vi "App3_measure_voltage_battery.vi"() -> ()   [LabVIEW 2015]
uses:
  <vilib>/DAQmx/read.llb/DAQmx Read (Analog DBL 1Chan 1Samp).vi
  <vilib>/DAQmx/read.llb/DAQmx Read (Analog Wfm 1Chan NSamp).vi
  <vilib>/DAQmx/miscellaneous.llb/DAQmx Fill In Error Info.vi
panel:
  out "error out":errorcluster
  in  "task out":refnum<k21>
  out "Button 2":u16
  out "Waveform Chart 2":waveform(dbl)
  out "Button":u16
  in  "Tab Control":T1(tab)
  out "min value":dbl
  out "max value":dbl
  out "Delta(s)":dbl
  in  "Zero":bool
  out "Average":dbl
  in  "mA/uA":bool
  out "Waveform Graph":waveform(dbl)(graph)
  in  "uA/mA":bool=TRUE
  out "Waveform Graph 2":waveform(dbl)(graph)
  out "Average (uA)":dbl caption="Average (mV)"
  in  "PAUSE":bool
  out "Vbat":dbl
  out "Waveform Chart":dbl(graph)
  in  "Number of samples uC Board":i32=10000
  in  "USB DAQ":tag="Dev1"
  out "Waveform Chart 3":dbl(graph)
  in  "file List":i32(listbox)
  out "2D Picture":picture
  # "FW Validation - Current Tracking V1.0"
  # "For uC Board: 20kS/s"
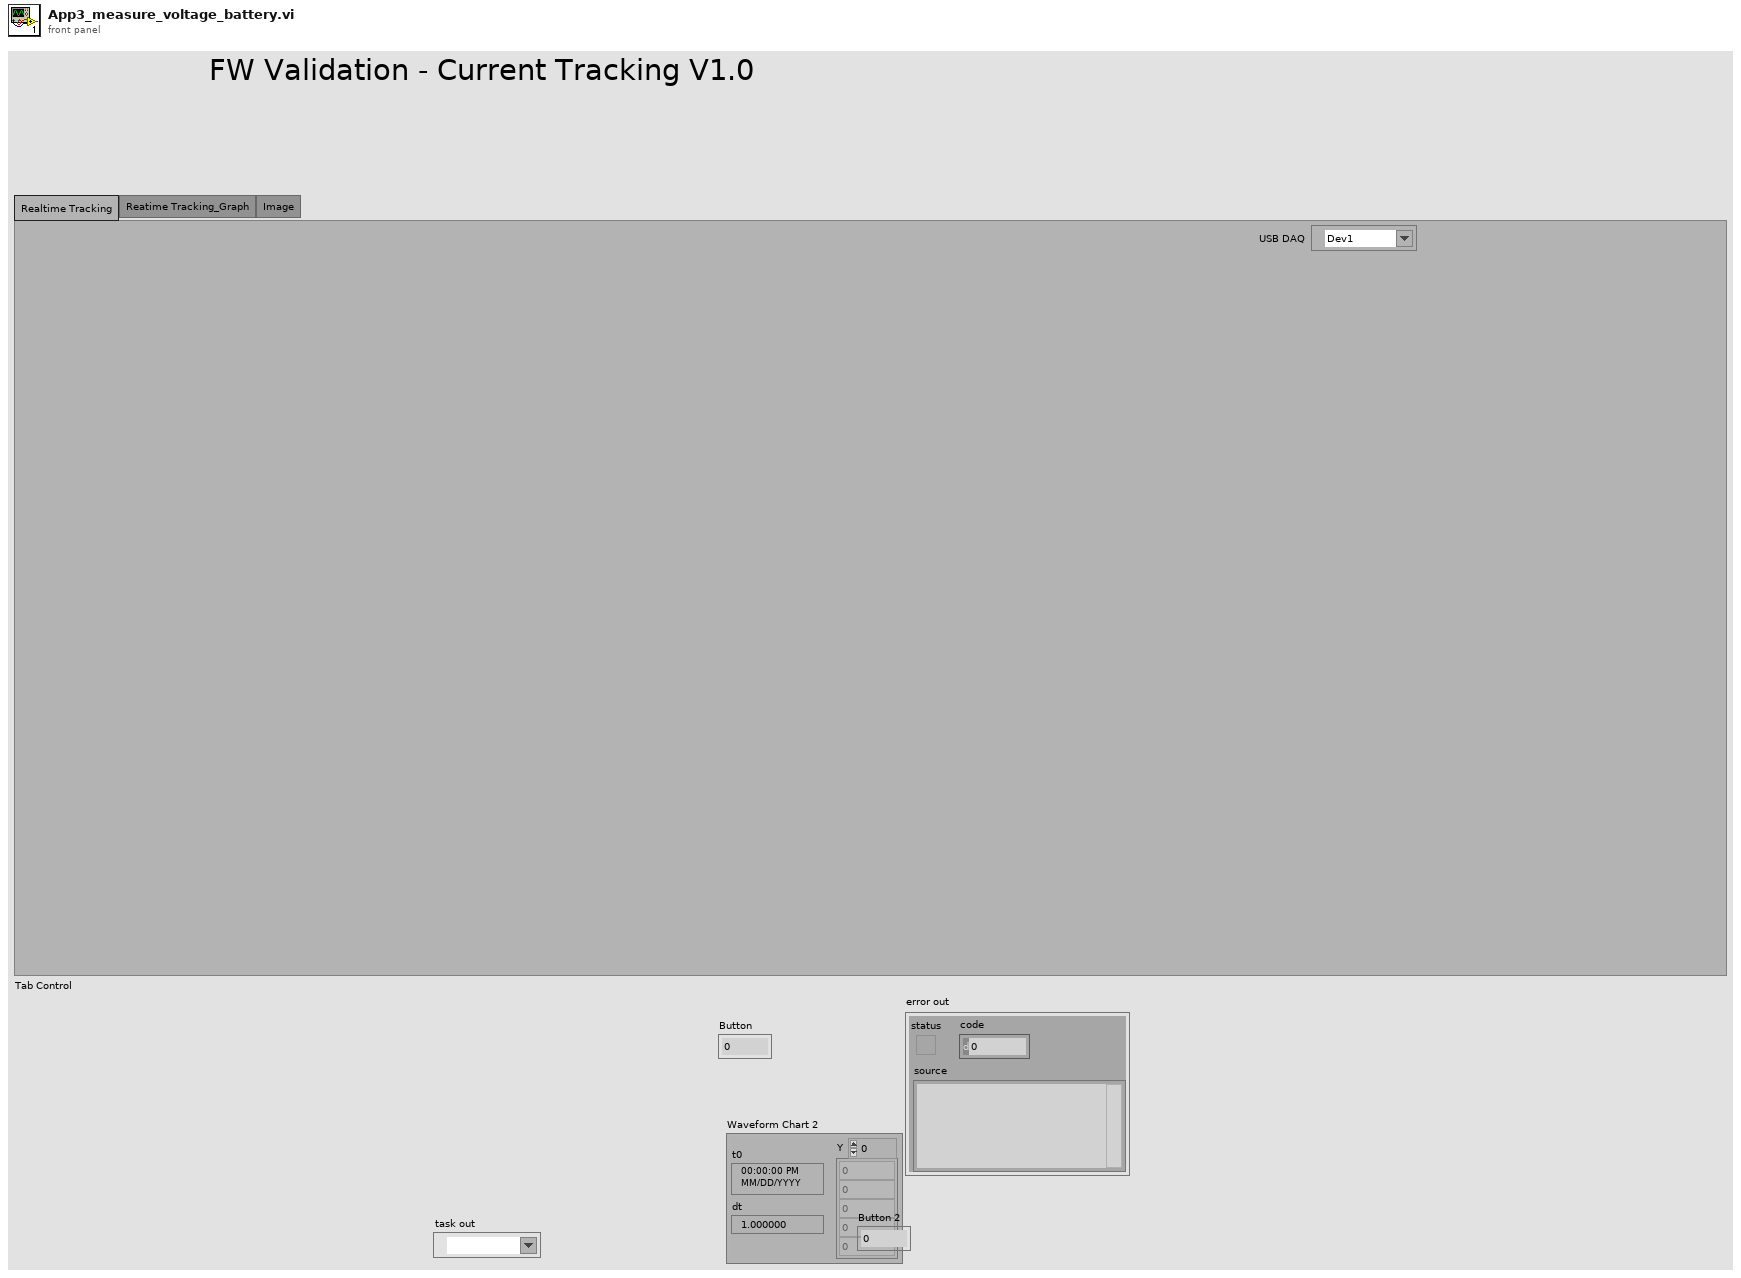
[diagram p1: front panel]
types:
  T1 = enum32{"Realtime Tracking", "Reatime Tracking_Graph", "Image"}
  T2 = typedef "imagedata.ctl" = cluster{"image type":i32, "image depth":i32, "image":u8[], "mask":u8[], "colors":u32[], "Rectangle":cluster{"left":i16, "top":i16, "right":i16, "bottom":i16}}
  T3 = typedef "LVCursorListTypeDef.ctl" = cluster{"Name":string, "Color":u32, "Style":u8, "Point Style":u8, "Name Visible":bool, "Allow Drag":bool, "Cursor Mode":u32, "Plot":i32, "Index":i32, "Position":cluster{"X":dbl, "Y":dbl}, "X Scale":u32, "Y Scale":u32, "Watch Plots":i32[], "Watch All Plots":bool, "Plot Area":i32, "Label Offset":cluster{"X":dbl, "Y":dbl}}[]
  T4 = cluster{"Name":string, "Color":u32, "Style":u8, "Point Style":u8, "Name Visible":bool, "Allow Drag":bool, "Cursor Mode":u32, "Plot":i32, "Index":i32, "Position":cluster{"X":dbl, "Y":dbl}, "X Scale":u32, "Y Scale":u32, "Watch Plots":i32[], "Watch All Plots":bool, "Plot Area":i32, "Label Offset":cluster{"X":dbl, "Y":dbl}}
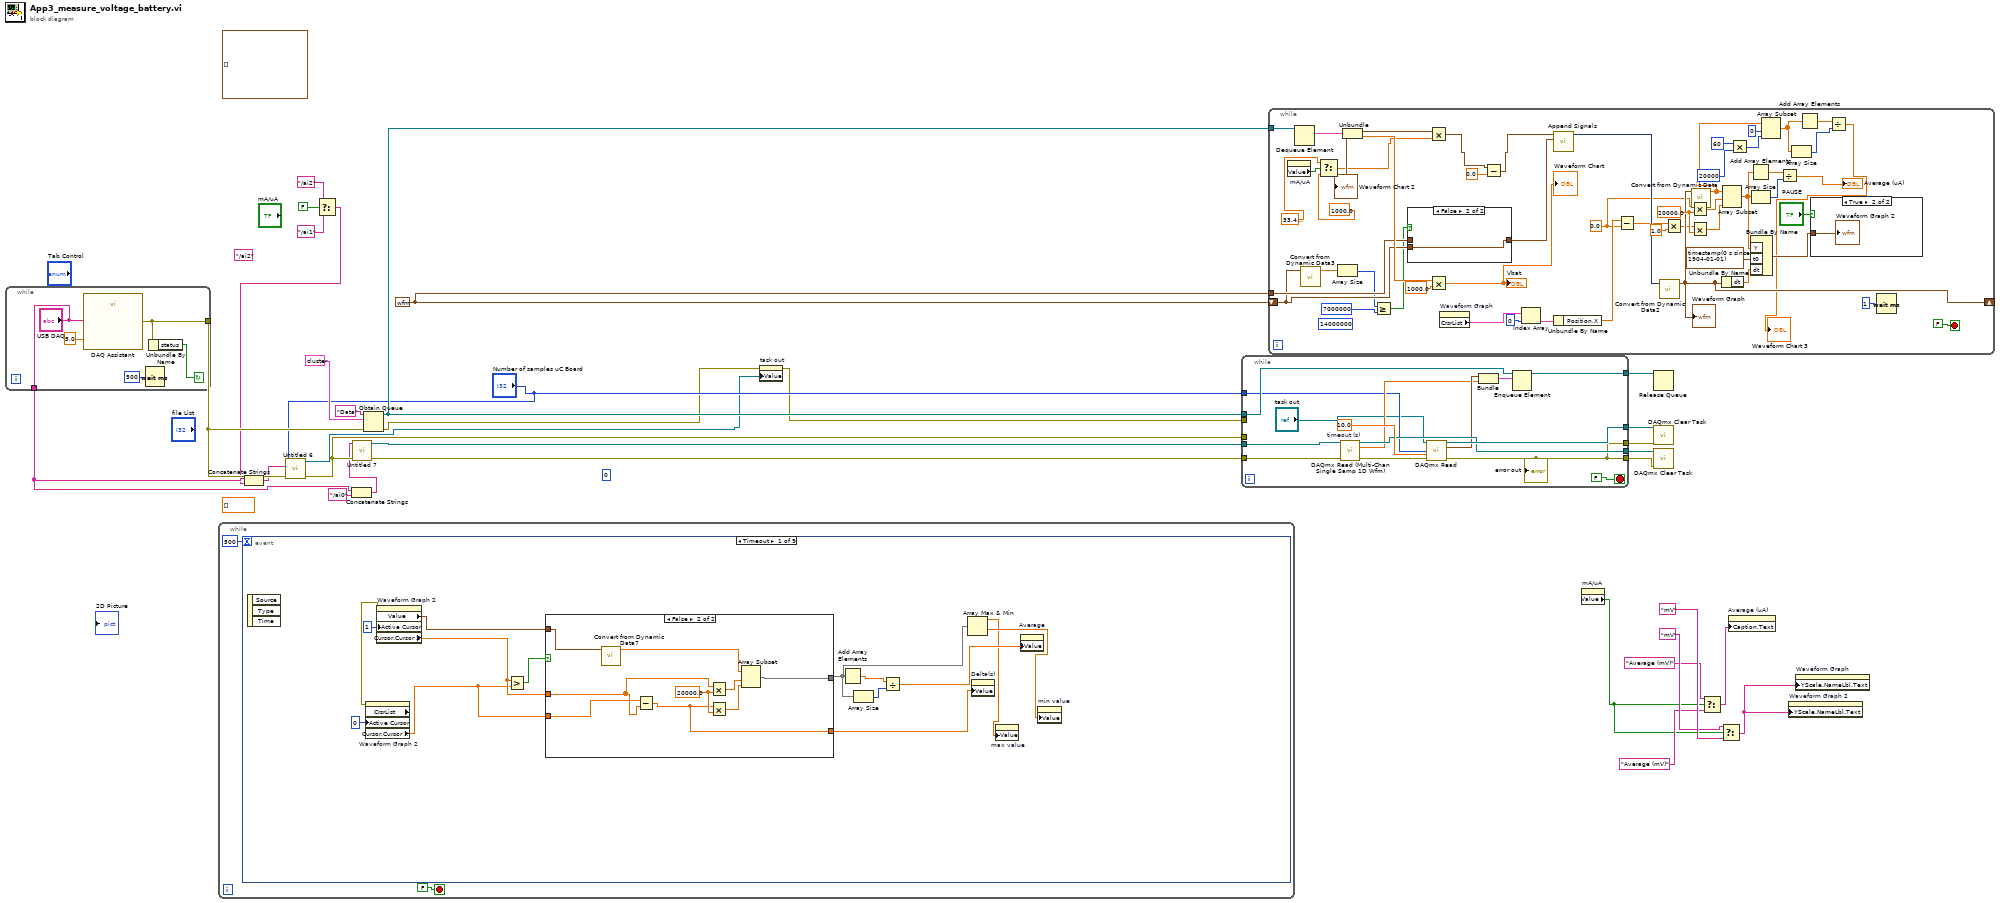
[diagram p0: block diagram]
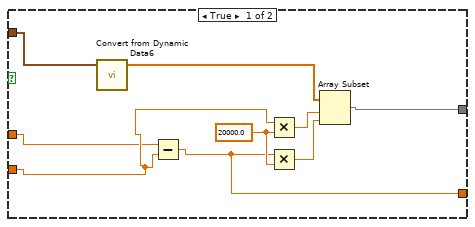
[diagram p2: hidden frame]
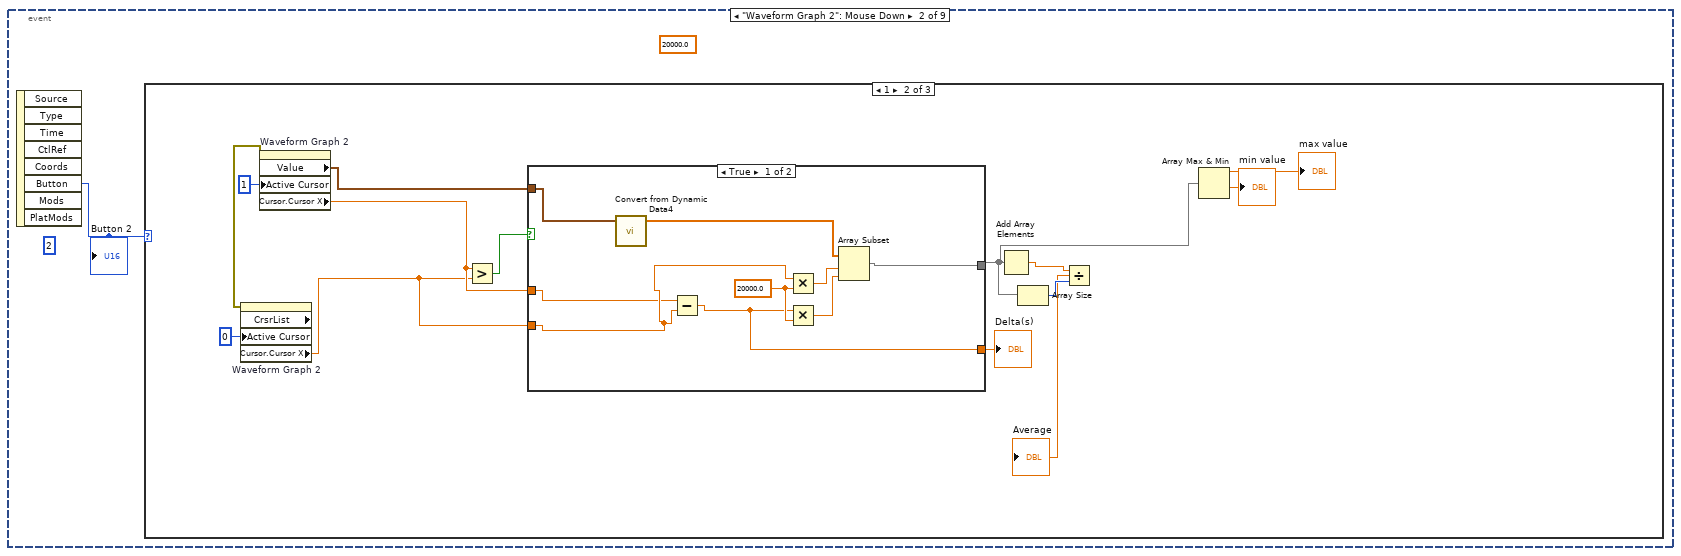
[diagram p3: hidden frame]
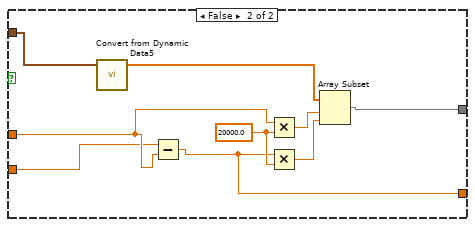
[diagram p5: hidden frame]
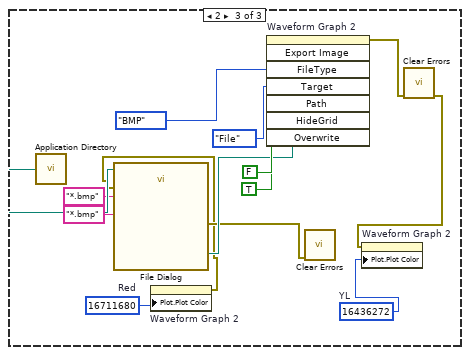
[diagram p6: hidden frame]
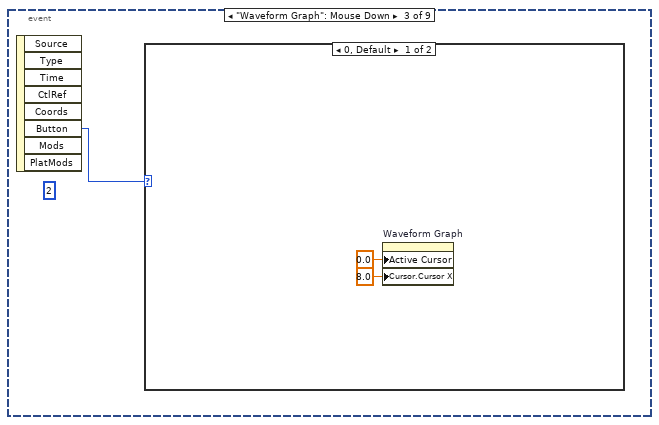
[diagram p7: hidden frame]
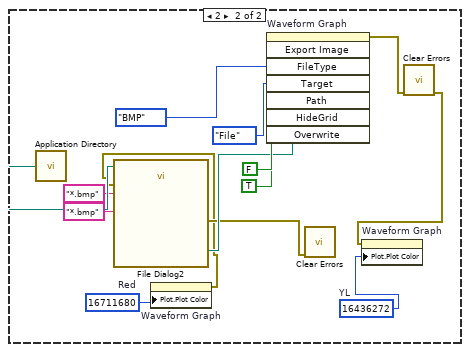
[diagram p8: hidden frame]
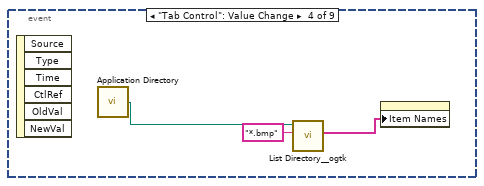
[diagram p9: hidden frame]
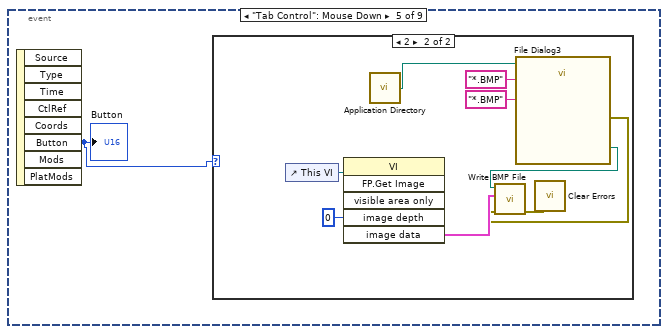
[diagram p10: hidden frame]
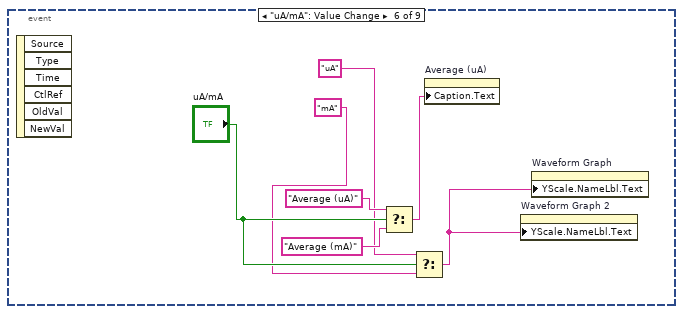
[diagram p12: hidden frame]
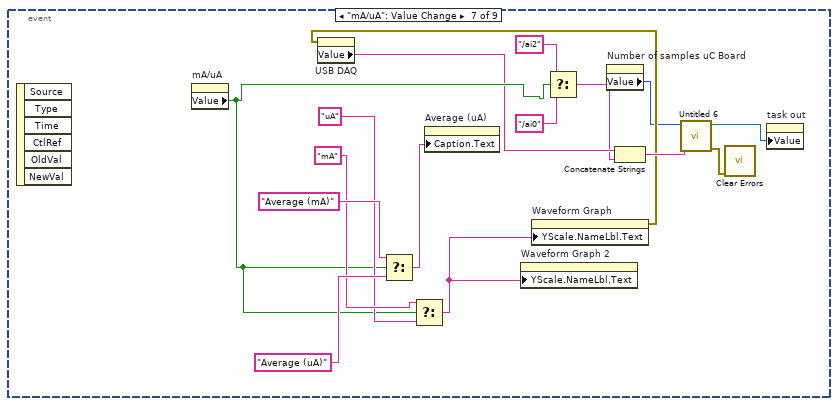
[diagram p13: hidden frame]
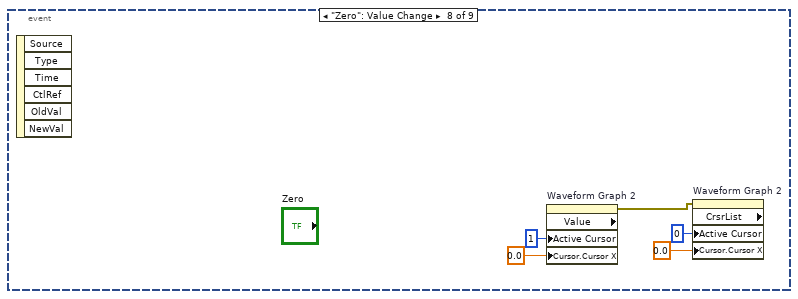
[diagram p14: hidden frame]
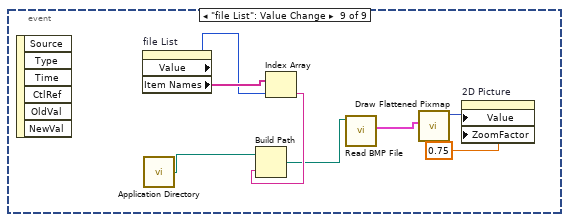
[diagram p15: hidden frame]
diagram:
  (unwired) u32 0 ("Active Cursor")
  (unwired) "/ai2" ("string")
  w20 = waveform(dbl) {"t0"=timestamp(0 s since 1904-01-01), "dt"=0.0, "Y"=[]} ("data")
  (unwired) waveform(dbl)[] [] ("History Data")
  (unwired) dbl[] [] ("Array")
  n1 = while {
    tunnel: [w35] -> w27
    tunnel: ["USB DAQ"] -> w17
    stop <- w34 continue-if-true
    n2 = call "DAQ Assistant"("data"=5.0, "device name"="USB DAQ") -> ("error out"=w35:errorcluster)  [unwired: 16 in, 1 out]
    n3 = Wait (ms)(milliseconds to wait=u32 500) -> ()  [unwired: 1 out]
    n4 = Unbundle By Name(w35) -> ("status"=w34:bool)
  }
  n5 = while {
    stop <- FALSE stop-if-true
    n6 = event shown="[0] Timeout" {
      selector: _ -> [_ _ _ _ _ _ _ _ _]
      dyn-events: _ -> [_ _ _ _ _ _ _ _ _]
      timeout: 500 -> [_ _ _ _ _ _ _ _ _]
      event Timeout {
        n7 = event-data() -> ()  [unwired: 1 in, 3 out]
        n8 = property on="Waveform Graph 2" class="WFGraph (strict)"("Active Cursor"=u32 1) -> (error out=w48:errorcluster, "Value"=w44:waveform(dbl), "Cursor.Cursor X"=w50:dbl)  [unwired: 2 in, 1 out]
        n9 = property on="Waveform Graph 2" class="WFGraph (strict)" props=["CrsrList", "Active Cursor", "Cursor", "Cursor X"](error in=w48, "Active Cursor"=u32 0) -> ("Cursor.Cursor X"=w49:dbl)  [unwired: 1 in, 3 out]
        n10 = Greater?(x=w50, y=w49) -> (0:w51:bool)
        n11 = case shown="False" w51 {
          tunnel: w44 -> [w62 w71]
          tunnel: w50 -> [w55 w65]
          tunnel: w49 -> [w56 w64]
          tunnel: [w57 w66] -> w45
          tunnel: [w54 w63] -> w43
          frame True {
            w60 = 20000.0 ("y")
            n12 = call "Convert from Dynamic Data6"("Dynamic Data Type"=w62) -> ("Array"=w58:dbl[])  [unwired: 3 in]
            n13 = Subtract(x=w55, y=w56) -> (x-y=w54:dbl)
            n14 = Multiply(x=w56, y=w60) -> (x*y=w61:dbl)
            n15 = Multiply(x=w54, y=w60) -> (x*y=w59:dbl)
            n16 = Array Subset(array=w58, index=w61, length=w59) -> (w57:dbl[])
          }
          frame False {
            w69 = 20000.0 ("y")
            n17 = call "Convert from Dynamic Data7"("Dynamic Data Type"=w71) -> ("Array"=w67:dbl[])  [unwired: 3 in]
            n18 = Subtract(x=w64, y=w65) -> (x-y=w63:dbl)
            n19 = Multiply(x=w65, y=w69) -> (x*y=w70:dbl)
            n20 = Multiply(x=w63, y=w69) -> (x*y=w68:dbl)
            n21 = Array Subset(array=w67, index=w70, length=w68) -> (w66:dbl[])
          }
        }
        n22 = Add Array Elements(numeric array=w45) -> (sum=w47:dbl)
        n23 = Array Size(array=w45) -> (size(s)=w46:i32)
        n24 = Divide(x=w47, y=w46) -> (x/y=w42:dbl)
        n25 = Array Max & Min(array=w45) -> (max value=w40:dbl, min value=w41:dbl)  [unwired: 2 out]
        n26 = property on="Delta(s)" class="DigNum (strict)"("Value"=w43) -> ()  [unwired: 2 in, 2 out]
        n27 = property on="max value" class="DigNum (strict)"("Value"=w40) -> ()  [unwired: 2 in, 2 out]
        n28 = property on="Average" class="DigNum (strict)"("Value"=w42) -> ()  [unwired: 2 in, 2 out]
        n29 = property on="min value" class="DigNum (strict)"("Value"=w41) -> ()  [unwired: 2 in, 2 out]
      }
      event "Waveform Graph 2": Mouse Down {
        (unwired) 20000.0 ("y")
        (unwired) u16 2 ("Button")
        n30 = event-data() -> ("Button"=w72:u16)  [unwired: 1 in, 7 out]
        "Button 2" <- w72
        n31 = case shown="1" w72 {
          frame 0, Default {
          }
          frame 1 {
            n32 = property on="Waveform Graph 2" class="WFGraph (strict)"("Active Cursor"=u32 1) -> (error out=w81:errorcluster, "Value"=w73:waveform(dbl), "Cursor.Cursor X"=w83:dbl)  [unwired: 2 in, 1 out]
            n33 = property on="Waveform Graph 2" class="WFGraph (strict)" props=["CrsrList", "Active Cursor", "Cursor", "Cursor X"](error in=w81, "Active Cursor"=u32 0) -> ("Cursor.Cursor X"=w82:dbl)  [unwired: 1 in, 3 out]
            n34 = Greater?(x=w83, y=w82) -> (0:w84:bool)
            n35 = case shown="True" w84 {
              tunnel: w73 -> [w95 w104]
              tunnel: w83 -> [w88 w98]
              tunnel: w82 -> [w89 w97]
              tunnel: [w90 w99] -> w76
              tunnel: [w87 w96] -> w77
              frame True {
                w93 = 20000.0 ("y")
                n36 = call "Convert from Dynamic Data4"("Dynamic Data Type"=w95) -> ("Array"=w91:dbl[])  [unwired: 3 in]
                n37 = Subtract(x=w88, y=w89) -> (x-y=w87:dbl)
                n38 = Multiply(x=w89, y=w93) -> (x*y=w94:dbl)
                n39 = Multiply(x=w87, y=w93) -> (x*y=w92:dbl)
                n40 = Array Subset(array=w91, index=w94, length=w92) -> (w90:dbl[])
              }
              frame False {
                w102 = 20000.0 ("y")
                n41 = call "Convert from Dynamic Data5"("Dynamic Data Type"=w104) -> ("Array"=w100:dbl[])  [unwired: 3 in]
                n42 = Subtract(x=w97, y=w98) -> (x-y=w96:dbl)
                n43 = Multiply(x=w98, y=w102) -> (x*y=w103:dbl)
                n44 = Multiply(x=w96, y=w102) -> (x*y=w101:dbl)
                n45 = Array Subset(array=w100, index=w103, length=w101) -> (w99:dbl[])
              }
            }
            "Delta(s)" <- w77
            n46 = Add Array Elements(numeric array=w76) -> (sum=w80:dbl)
            n47 = Array Size(array=w76) -> (size(s)=w79:i32)
            n48 = Divide(x=w80, y=w79) -> (x/y=→"Average":dbl)
            n49 = Array Max & Min(array=w76) -> (max value=→"max value":dbl, min value=→"min value":dbl)  [unwired: 2 out]
          }
          frame 2 {
            w105 = u32 16436272  # YL
            w107 = u32 16711680  # Red
            n50 = call <vilib>:"Application Directory.vi"() -> ("Application Directory"=w114:path)
            n51 = property on="Waveform Graph 2" class="WFGraph (strict)"("Plot.Plot Color"=w107) -> (error out=w108:errorcluster)  [unwired: 2 in, 1 out]
            n52 = call "File Dialog"("start path"=w114, "error in"=w108, "pattern (all files)"="*.bmp", "pattern label"="*.bmp") -> ("selected path"=w111:path, "error out"=w110:errorcluster)  [unwired: 8 in, 2 out]
            n53 = invoke on="Waveform Graph 2" class="WFGraph (strict)" method="Export Image"("FileType"=enum32{"BMP", "EPS", "EMF", "PICT"}."BMP" ("File Type"), "Target"=enum32{"File", "Clipboard"}."File", "Path"=w111, "HideGrid"=FALSE ("Hide Grid"), "Overwrite"=TRUE ("Always Overwrite")) -> (error out=w109:errorcluster)  [unwired: 3 in, 7 out]
            n54 = call <vilib>:"Clear Errors.vi"("error in (no error)"=w110) -> ()  [unwired: 5 in, 2 out]
            n55 = call <vilib>:"Clear Errors.vi"("error in (no error)"=w109) -> ("error out"=w106:errorcluster)  [unwired: 5 in, 1 out]
            n56 = property on="Waveform Graph 2" class="WFGraph (strict)"(error in=w106, "Plot.Plot Color"=w105) -> ()  [unwired: 1 in, 2 out]
          }
        }
      }
      event "Waveform Graph": Mouse Down {
        (unwired) u16 2 ("Button")
        n57 = event-data() -> ("Button"=w119:u16)  [unwired: 1 in, 7 out]
        n58 = case shown="0, Default" w119 {
          frame 0, Default {
            n59 = property on="Waveform Graph" class="WFGraph (strict)"("Active Cursor"=0.0 ("Cursor.Cursor Position:Cursor X"), "Cursor.Cursor X"=8.0 ("Cursor.Cursor Position:Cursor X")) -> ()  [unwired: 2 in, 2 out]
          }
          frame 2 {
            w122 = u32 16436272  # YL
            w124 = u32 16711680  # Red
            n60 = call <vilib>:"Application Directory.vi"() -> ("Application Directory"=w131:path)
            n61 = property on="Waveform Graph" class="WFGraph (strict)"("Plot.Plot Color"=w124) -> (error out=w125:errorcluster)  [unwired: 2 in, 1 out]
            n62 = call "File Dialog2"("start path"=w131, "error in"=w125, "pattern (all files)"="*.bmp", "pattern label"="*.bmp") -> ("selected path"=w128:path, "error out"=w127:errorcluster)  [unwired: 8 in, 2 out]
            n63 = invoke on="Waveform Graph" class="WFGraph (strict)" method="Export Image"("FileType"=enum32{"BMP", "EPS", "EMF", "PICT"}."BMP" ("File Type"), "Target"=enum32{"File", "Clipboard"}."File", "Path"=w128, "HideGrid"=FALSE ("Hide Grid"), "Overwrite"=TRUE ("Always Overwrite")) -> (error out=w126:errorcluster)  [unwired: 3 in, 7 out]
            n64 = call <vilib>:"Clear Errors.vi"("error in (no error)"=w127) -> ()  [unwired: 5 in, 2 out]
            n65 = call <vilib>:"Clear Errors.vi"("error in (no error)"=w126) -> ("error out"=w123:errorcluster)  [unwired: 5 in, 1 out]
            n66 = property on="Waveform Graph" class="WFGraph (strict)"(error in=w123, "Plot.Plot Color"=w122) -> ()  [unwired: 1 in, 2 out]
          }
        }
      }
      event "Tab Control": Value Change {
        n67 = event-data() -> ()  [unwired: 1 in, 6 out]
        n68 = call <vilib>:"Application Directory.vi"() -> ("Application Directory"=w138:path)
        n69 = call <userlib>:"List Directory__ogtk.vi"("pattern"="*.bmp", "directory path"=w138) -> ("file names"=w136:string[])  [unwired: 2 in, 3 out]
        n70 = property on="file List" class="LstBox (strict)"("Item Names"=w136) -> ()  [unwired: 2 in, 2 out]
      }
      event "Tab Control": Mouse Down {
        n71 = event-data() -> ("Button"=w139:u16)  [unwired: 1 in, 7 out]
        "Button" <- w139
        n72 = case shown="2" w139 {
          frame 0, Default {
          }
          frame 2 {
            n73 = control-ref of="This VI"() -> (w148:refnum<vi>)
            n74 = invoke class="VI" method="FP.Get Image"(reference=w148, "image depth"=0 ("Image Depth")) -> ("image data"=w146:T2)  [unwired: 4 in, 5 out]
            n75 = call <vilib>:"Application Directory.vi"() -> ("Application Directory"=w142:path)
            n76 = call "File Dialog3"("start path"=w142, "pattern (all files)"="*.BMP", "pattern label"="*.BMP") -> ("selected path"=w145:path, "error out"=w144:errorcluster)  [unwired: 9 in, 2 out]
            n77 = call <vilib>:"Write BMP File.vi"("error in (no error)"=w144, "image data"=w146, "path to BMP file"=w145) -> ("error out"=w140:errorcluster)  [unwired: 7 in, 1 out]
            n78 = call <vilib>:"Clear Errors.vi"("error in (no error)"=w140) -> ()  [unwired: 5 in, 2 out]
          }
        }
      }
      event "uA/mA": Value Change {
        n79 = event-data() -> ()  [unwired: 1 in, 6 out]
        n80 = Select(t="Average (uA)" ("Caption.Text"), s="uA/mA", f="Average (mA)" ("Caption.Text")) -> (s? t:f=w155:string)
        n81 = Select(t="uA" ("Caption.Text"), s="uA/mA", f="mA" ("Caption.Text")) -> (s? t:f=w149:string)
        n82 = property on="Average (uA)" class="DigNum (strict)"("Caption.Text"=w155) -> ()  [unwired: 2 in, 2 out]
        n83 = property on="Waveform Graph 2" class="WFGraph (strict)"("YScale.NameLbl.Text"=w149) -> ()  [unwired: 2 in, 2 out]
        n84 = property on="Waveform Graph" class="WFGraph (strict)"("YScale.NameLbl.Text"=w149) -> ()  [unwired: 2 in, 2 out]
      }
      event "mA/uA": Value Change {
        n85 = event-data() -> ()  [unwired: 1 in, 6 out]
        n86 = property on="mA/uA" class="Bool (strict)"() -> ("Value"=w163:bool)  [unwired: 2 in, 2 out]
        n87 = Select(t="Average (mA)" ("Caption.Text"), s=w163, f="Average (uA)" ("Caption.Text")) -> (s? t:f=w171:string)
        n88 = Select(t="mA" ("Caption.Text"), s=w163, f="uA" ("Caption.Text")) -> (s? t:f=w170:string)
        n89 = property on="Average (uA)" class="DigNum (strict)"("Caption.Text"=w171) -> ()  [unwired: 2 in, 2 out]
        n90 = property on="Waveform Graph 2" class="WFGraph (strict)"("YScale.NameLbl.Text"=w170) -> ()  [unwired: 2 in, 2 out]
        n91 = property on="Waveform Graph" class="WFGraph (strict)"("YScale.NameLbl.Text"=w170) -> (error out=w159:errorcluster)  [unwired: 2 in, 1 out]
        n92 = property on="USB DAQ" class="DAQmxName"(error in=w159) -> ("Value"=w161:string)  [unwired: 1 in, 2 out]
        n93 = Select(t="/ai2" ("string"), s=w163, f="/ai0" ("string")) -> (s? t:f=w160:string)
        n94 = property on="Number of samples uC Board" class="DigNum (strict)"() -> ("Value"=w158:i32)  [unwired: 2 in, 2 out]
        n95 = Concatenate Strings(w161, w160) -> (w162:string)
        n96 = call "Untitled 6.vi"("physical channel"=w162, "number of samples"=w158) -> ("error out"=w156:errorcluster, "task out"=w157:refnum<k21>)  [unwired: 8 in]
        n97 = call <vilib>:"Clear Errors.vi"("error in (no error)"=w156) -> ()  [unwired: 5 in, 2 out]
        n98 = property on="task out" class="DAQmxName (strict)"("Value"=w157) -> ()  [unwired: 2 in, 2 out]
      }
      event "Zero": Value Change {
        n99 = event-data() -> ()  [unwired: 1 in, 6 out]
        n100 = property on="Waveform Graph 2" class="WFGraph (strict)" props=["Value", "Active Cursor", "Cursor", "Cursor X"]("Active Cursor"=u32 1, "Cursor.Cursor X"=0.0 ("Cursor.Cursor Position:Cursor X")) -> (error out=w174:errorcluster)  [unwired: 2 in, 2 out]
        n101 = property on="Waveform Graph 2" class="WFGraph (strict)" props=["CrsrList", "Active Cursor", "Cursor", "Cursor X"](error in=w174, "Active Cursor"=u32 0, "Cursor.Cursor X"=0.0 ("Cursor.Cursor Position:Cursor X")) -> ()  [unwired: 1 in, 3 out]
      }
      event "file List": Value Change {
        n102 = event-data() -> ()  [unwired: 1 in, 6 out]
        n103 = property on="file List" class="LstBox (strict)"() -> ("Value"=w183:i32, "Item Names"=w184:string[])  [unwired: 2 in, 2 out]
        n104 = call <vilib>:"Application Directory.vi"() -> ("Application Directory"=w180:path)
        n105 = Index Array(array=w184, index=w183) -> (element=w179:string)
        n106 = Build Path(base path=w180, name or relative path=w179) -> (appended path=w178:path)
        n107 = call <vilib>:"Read BMP File.vi"("path to BMP file"=w178) -> ("image data"=w182:T2)  [unwired: 8 in, 2 out]
        n108 = call <vilib>:"Draw Flattened Pixmap.vi"("image data"=w182) -> ("new picture"=w181:picture)  [unwired: 8 in]
        n109 = property on="2D Picture" class="Pict"("Value"=w181, "ZoomFactor"=sgl 0.75 ("Zoom Factor")) -> ()  [unwired: 2 in, 2 out]
      }
    }
  }
  n110 = Select(t="/ai2" ("string"), s=FALSE, f="/ai1" ("string")) -> (s? t:f=w12:string)
  n111 = Concatenate Strings(w17, w12) -> (w18:string)
  n112 = call "Untitled 6.vi"("error in"=w27, "physical channel"=w18, "number of samples"="Number of samples uC Board") -> ("error out"=w22:errorcluster, "task out"=w4:refnum<k21>)  [unwired: 7 in]
  n113 = Concatenate Strings(w17, "/ai0" ("string")) -> (w15:string)
  n114 = call "Untitled 7.vi"("error in"=w22, "physical channel"=w15) -> ("error out"=w25:errorcluster, "task out"=w26:refnum<k21>)  [unwired: 8 in]
  n115 = Obtain Queue(name (unnamed)="Data", element data type=cluster{"Waveform Chart 2":waveform(dbl), dbl} {"Waveform Chart 2"={"t0"=timestamp(0 s since 1904-01-01), "dt"=1.0, "Y"=[]}, 0.0}, error in (no error)=w27) -> (queue out=w29:refnum<queue>, error out=w3:errorcluster)  [unwired: 2 in, 1 out]
  n116 = property on="task out" class="DAQmxName (strict)"(error in=w3, "Value"=w4) -> (error out=w2:errorcluster)  [unwired: 1 in, 1 out]
  n117 = while {
    tunnel: w22 -> [_]
    tunnel: [w199] -> w32
    tunnel: [w190] -> w31
    tunnel: w29 -> [w197]
    tunnel: [w196] -> w28
    tunnel: w26 -> [w194]
    tunnel: w25 -> [w193]
    tunnel: [w192] -> w24
    tunnel: [w190] -> w23
    tunnel: "Number of samples uC Board" -> [w186]
    tunnel: w2 -> [_]
    stop <- FALSE ("stop (F)") stop-if-true
    w198 = 10.0  # timeout (s)
    n118 = call-poly "DAQmx Read (Multi-Chan Single Samp 1D Wfm).vi"("task/channels in"=w194, "error in"=w193) -> ("task out"=w192:refnum<k21>, "data"=w188:dbl, "error out"=w191:errorcluster)  [unwired: 11 in]
    n119 = call-poly <vilib>:"DAQmx Read.vi"("task/channels in"="task out", "number of samples per channel"=w186, "timeout"=w198, "error in"=w191) -> ("task out"=w199:refnum<k21>, "data"=w189:waveform(dbl), "error out"=w190:errorcluster)  [unwired: 9 in]
    "error out" <- w190
    n120 = Bundle("data"=w189, "data"=w188) -> (w187:cluster{"data":waveform(dbl), "data":dbl})  [unwired: 1 in]
    n121 = Enqueue Element(queue=w197, element=w187) -> (queue out=w196:refnum<queue>)  [unwired: 2 in, 2 out]
  }
  n122 = while {
    tunnel: w29 -> [w251]
    shift-right: [w240] -> _
    shift-left: w20 -> [w220]
    tunnel: w20 -> [w221]
    stop <- FALSE stop-if-true
    (unwired) 14000000 ("size(s)")
    w230 = 0.0
    w244 = 20000.0 ("y")
    n123 = property on="mA/uA" class="Bool (strict)"() -> ("Value"=w212:bool)  [unwired: 2 in, 2 out]
    n124 = Dequeue Element(queue=w251) -> (element=w227:cluster{"Waveform Chart 2":waveform(dbl), dbl})  [unwired: 2 in, 3 out]
    n125 = call "Convert from Dynamic Data3"("Dynamic Data Type"=w220) -> ("Array"=w219:dbl[])  [unwired: 3 in]
    n126 = Select(t=33.499999999999986 ("y"), s=w212, f=1000.0 ("y")) -> (s? t:f=w209:dbl)
    n127 = Array Size(array=w219) -> (size(s)=w218:i32)
    n128 = Unbundle(w227) -> ("Waveform Chart 2"=w226:waveform(dbl), w225:dbl)
    "Waveform Chart 2" <- w226
    n129 = Greater Or Equal?(x=w218, y=7000000 ("size(s)")) -> (x >= y?=w216:bool)
    n130 = case shown="False" w216 {
      tunnel: w220 -> [_ w253]
      tunnel: [w252 w253] -> w222
      tunnel: w221 -> [w252 _]
      frame True {
      }
      frame False {
      }
    }
    n131 = Multiply(x=w226, y=w209) -> (x*y=w213:waveform(dbl))
    n132 = Multiply(x=w225, y=1000.0) -> (x*y=→"Vbat" →"Waveform Chart":dbl)
    n133 = property on="Waveform Graph" class="WFGraph (strict)"() -> ("CrsrList"=w247:T3)  [unwired: 2 in, 2 out]
    n134 = Subtract(x=w213, y=0.0) -> (x-y=w214:waveform(dbl))
    n135 = Index Array(array=w247, index=0) -> (element=w228:T4)
    n136 = call "Append Signals"("Input Signal B"=w222, "Input Signal A"=w214) -> ("Appended Signals"=w248:dynamicdata)  [unwired: 8 in, 1 out]
    n137 = Unbundle By Name(w228) -> ("Position.X"=w231:dbl)
    n138 = Subtract(x=w231, y=w230) -> (x-y=w234:dbl)
    n139 = call "Convert from Dynamic Data2"("Dynamic Data Type"=w248) -> ("Waveform"=w240:waveform(dbl))  [unwired: 3 in]
    "Waveform Graph" <- w240
    n140 = Multiply(x=w234, y=1.0) -> (x*y=w232:dbl)
    n141 = Multiply(x=w230, y=w244) -> (x*y=w245:dbl)
    n142 = Multiply(x=w232, y=w244) -> (x*y=w243:dbl)
    n143 = call "Convert from Dynamic Data"("Dynamic Data Type"=w240) -> ("Array"=w207:dbl[])  [unwired: 3 in]
    n144 = Unbundle By Name(w240) -> ("dt"=w239:dbl)
    n145 = Array Subset(array=w207, index=w245, length=w243) -> (w238:dbl[])
    n146 = Multiply(x=60, y=20000) -> (x*y=w203:i32)
    n147 = Add Array Elements(numeric array=w238) -> (sum=w237:dbl)
    n148 = Bundle By Name("Y"=w238, "t0"=timestamp(0 s since 1904-01-01), "dt"=w239) -> (w242:waveform(dbl))  [unwired: 1 in]
    n149 = Array Size(array=w238) -> (size(s)=w236:i32)
    n150 = Array Subset(array=w207, index=0, length=w203) -> (w206:dbl[])
    n151 = Divide(x=w237, y=w236) -> (x/y=→"Average (uA)":dbl)
    n152 = Array Size(array=w206) -> (size(s)=w205:i32)
    n153 = Add Array Elements(numeric array=w206) -> (sum=w208:dbl)
    n154 = case shown="True" "PAUSE" {
      tunnel: w242 -> [_ w254]
      frame False {
      }
      frame True {
        "Waveform Graph 2" <- w254
      }
    }
    n155 = Divide(x=w208, y=w205) -> (x/y=→"Waveform Chart 3":dbl)
    n156 = Wait (ms)(milliseconds to wait=u32 1) -> ()  [unwired: 1 out]
  }
  n157 = property on="mA/uA" class="Bool (strict)"() -> ("Value"=w7:bool)  [unwired: 2 in, 2 out]
  n158 = Release Queue(queue=w28) -> ()  [unwired: 2 in, 3 out]
  n159 = call <vilib>:"DAQmx Clear Task.vi"("task in"=w32, "error in"=w31) -> ()  [unwired: 13 in, 1 out]
  n160 = call <vilib>:"DAQmx Clear Task.vi"("task in"=w24, "error in"=w23) -> ()  [unwired: 13 in, 1 out]
  n161 = Select(t="Average (mV)" ("Caption.Text"), s=w7, f="Average (mV)" ("Caption.Text")) -> (s? t:f=w5:string)
  n162 = Select(t="mV" ("Caption.Text"), s=w7, f="mV" ("Caption.Text")) -> (s? t:f=w6:string)
  n163 = property on="Average (uA)" class="DigNum (strict)"("Caption.Text"=w5) -> ()  [unwired: 2 in, 2 out]
  n164 = property on="Waveform Graph 2" class="WFGraph (strict)"("YScale.NameLbl.Text"=w6) -> ()  [unwired: 2 in, 2 out]
  n165 = property on="Waveform Graph" class="WFGraph (strict)"("YScale.NameLbl.Text"=w6) -> ()  [unwired: 2 in, 2 out]
